vi "rx_ceEq.vi"(2 "preamble":cdb[](array[numeric])=[-0.7071067811865475+0.7071067811865476i, 0.7071067811865476+0.7071067811865475i, 0.7071067811865474-0.7071067811865477i, 0.7071067811865476+0.7071067811865475i, -0.7071067811865475+0.7071067811865476i, -0.7071067811865477-0.7071067811865475i, 0.7071067811865476+0.7071067811865475i, -0.7071067811865477-0.7071067811865475i, -0.7071067811865475+0.7071067811865476i, 0.7071067811865476+0.7071067811865475i, 0.7071067811865474-0.7071067811865477i, 0.7071067811865476+0.7071067811865475i, -0.7071067811865475+0.7071067811865476i, -0.7071067811865477-0.7071067811865475i, 0.7071067811865476+0.7071067811865475i, -0.7071067811865477-0.7071067811865475i, -0.7071067811865475+0.7071067811865476i, 0.7071067811865476+0.7071067811865475i, 0.7071067811865474-0.7071067811865477i, 0.7071067811865476+0.7071067811865475i, -0.7071067811865475+0.7071067811865476i, -0.7071067811865477-0.7071067811865475i, 0.7071067811865476+0.7071067811865475i, -0.7071067811865477-0.7071067811865475i, -0.7071067811865475+0.7071067811865476i, 0.7071067811865476+0.7071067811865475i, 0.7071067811865474-0.7071067811865477i, 0.7071067811865476+0.7071067811865475i, -0.7071067811865475+0.7071067811865476i, -0.7071067811865477-0.7071067811865475i, 0.7071067811865476+0.7071067811865475i, -0.7071067811865477-0.7071067811865475i, -0.7071067811865475+0.7071067811865476i, 0.7071067811865476+0.7071067811865475i, 0.7071067811865474-0.7071067811865477i, 0.7071067811865476+0.7071067811865475i, -0.7071067811865475+0.7071067811865476i, -0.7071067811865477-0.7071067811865475i, 0.7071067811865476+0.7071067811865475i, -0.7071067811865477-0.7071067811865475i, -0.7071067811865475+0.7071067811865476i, 0.7071067811865476+0.7071067811865475i, 0.7071067811865474-0.7071067811865477i, 0.7071067811865476+0.7071067811865475i, -0.7071067811865475+0.7071067811865476i, -0.7071067811865477-0.7071067811865475i, 0.7071067811865476+0.7071067811865475i, -0.7071067811865477-0.7071067811865475i, -0.7071067811865475+0.7071067811865476i, 0.7071067811865476+0.7071067811865475i, 0.7071067811865474-0.7071067811865477i, 0.7071067811865476+0.7071067811865475i, -0.7071067811865475+0.7071067811865476i, -0.7071067811865477-0.7071067811865475i, 0.7071067811865476+0.7071067811865475i, -0.7071067811865477-0.7071067811865475i, -0.7071067811865475+0.7071067811865476i, 0.7071067811865476+0.7071067811865475i, 0.7071067811865474-0.7071067811865477i, 0.7071067811865476+0.7071067811865475i, -0.7071067811865475+0.7071067811865476i, -0.7071067811865477-0.7071067811865475i, 0.7071067811865476+0.7071067811865475i, -0.7071067811865477-0.7071067811865475i], 3 "symbols":cdb[](array[numeric])) -> (0 "valid?":bool, 1 "eq symbols":cdb[](array[numeric]))   [LabVIEW 2014]
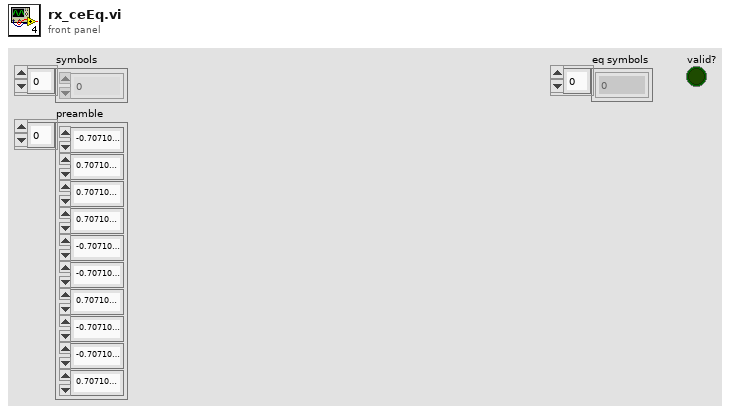
[diagram p1: front panel]
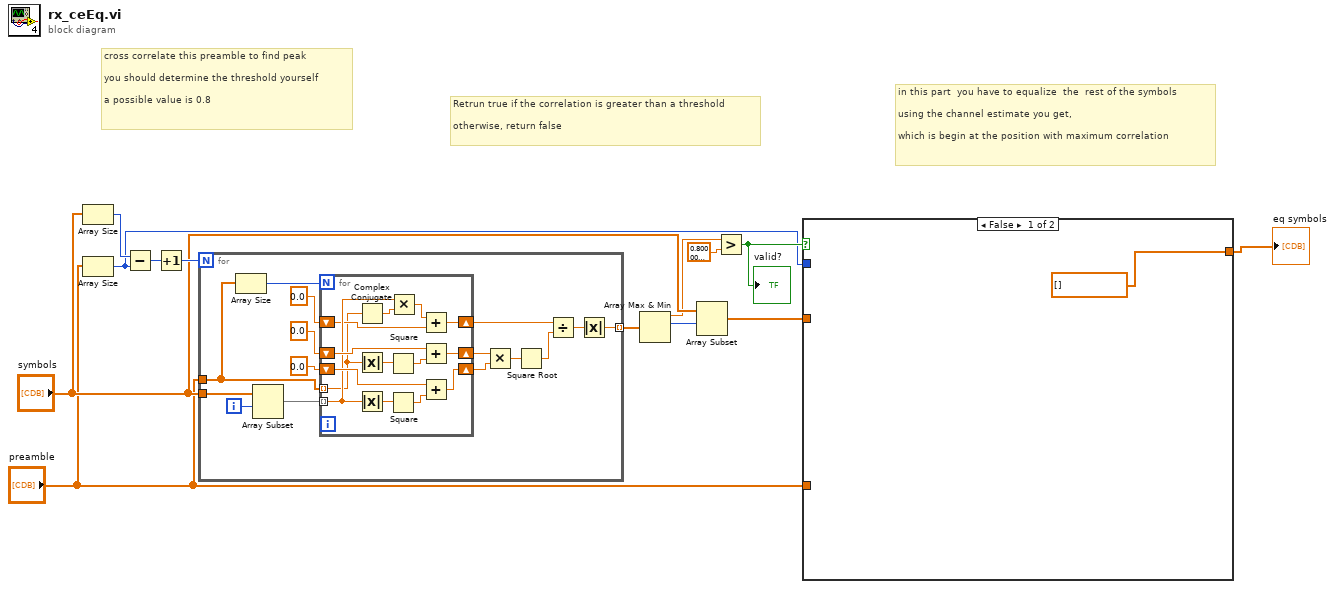
[diagram p0: block diagram]
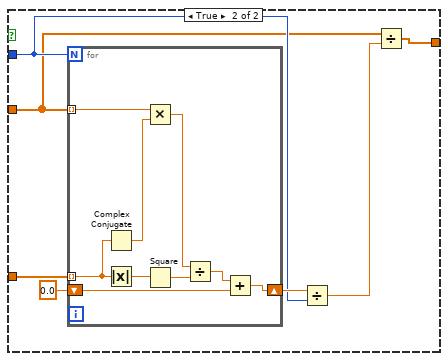
[diagram p2: hidden frame]
diagram:
  # "in this part  you have to equalize  the  rest of the symbols\n\nusing the channel estimate you get, \n\nwhich is begin at the position with maximum correlation"
  # "Retrun true if the correlation is greater than a threshold\n\notherwise, return false"
  # "cross correlate this preamble to find peak \n\nyou should determine the threshold yourself\n\na possible value is 0.8"
  n1 = Array Size(array="symbols") -> (size(s)=w10:i32)
  n2 = Array Size(array="preamble") -> (size(s)=w3:i32)
  n3 = Subtract(x=w10, y=w3) -> (x-y=w12:i32)
  n4 = Increment(x=w12) -> (x+1=w11:i32)
  n5 = for {
    N: w11 -> [_]
    tunnel: "preamble" -> [w27]
    tunnel: "symbols" -> [w26]
    tunnel: [w17] -> w7 mode=indexing
    i -> [w20]
    n6 = Array Size(array=w27) -> (size(s)=w28:i32)
    n7 = Array Subset(array=w26, index=w20) -> (w25:cdb[])  [unwired: 1 in]
    n8 = for {
      N: w28 -> [_]
      tunnel: w27 -> [w29] mode=indexing
      shift-right: [w39] -> w24
      shift-left: 0.0 -> [w41]
      shift-right: [w36] -> w23
      shift-left: 0.0 -> [w35]
      tunnel: w25 -> [w34] mode=indexing
      shift-right: [w30] -> w22
      shift-left: 0.0 -> [w31]
      n9 = Complex Conjugate(1:w29) -> (0:w33:cdb)
      n10 = Absolute Value(x=w29) -> (abs(x)=w42:dbl)
      n11 = Absolute Value(x=w34) -> (abs(x)=w38:dbl)
      n12 = Square(x=w42) -> (x^2=w40:dbl)
      n13 = Square(x=w38) -> (x^2=w37:dbl)
      n14 = Multiply(x=w34, y=w33) -> (x*y=w32:cdb)
      n15 = Add(x=w32, y=w31) -> (x+y=w30:cdb)
      n16 = Add(x=w41, y=w40) -> (x+y=w39:dbl)
      n17 = Add(x=w35, y=w37) -> (x+y=w36:dbl)
    }
    n18 = Multiply(x=w24, y=w23) -> (x*y=w19:dbl)
    n19 = Square Root(x=w19) -> (sqrt(x)=w18:dbl)
    n20 = Divide(x=w22, y=w18) -> (x/y=w21:cdb)
    n21 = Absolute Value(x=w21) -> (abs(x)=w17:dbl)
  }
  n22 = Array Max & Min(array=w7) -> (max value=w5:dbl, max index (indices)=w8:i32)  [unwired: 2 out]
  n23 = Array Subset(array="symbols", index=w8) -> (w2:cdb[])  [unwired: 1 in]
  n24 = Greater?(x=w5, y=sgl 0.8) -> (0:w4:bool)
  "valid?" <- w4
  n25 = case shown="False" w4 {
    tunnel: [cdb[] [] w50] -> w13
    tunnel: w3 -> [_ w46]
    tunnel: w2 -> [_ w45]
    tunnel: "preamble" -> [_ w47]
    frame False {
    }
    frame True {
      n26 = for {
        N: w46 -> [_]
        shift-right: [w52] -> w49
        shift-left: 0.0 -> [w54]
        tunnel: w45 -> [w57] mode=indexing
        tunnel: w47 -> [w51] mode=indexing
        n27 = Complex Conjugate(1:w51) -> (0:w59:cdb)
        n28 = Absolute Value(x=w51) -> (abs(x)=w58:dbl)
        n29 = Multiply(x=w57, y=w59) -> (x*y=w56:cdb)
        n30 = Square(x=w58) -> (x^2=w55:dbl)
        n31 = Divide(x=w56, y=w55) -> (x/y=w53:cdb)
        n32 = Add(x=w53, y=w54) -> (x+y=w52:cdb)
      }
      n33 = Divide(x=w49, y=w46) -> (x/y=w44:cdb)
      n34 = Divide(x=w45, y=w44) -> (x/y=w50:cdb[])
    }
  }
  "eq symbols" <- w13
